vi "fit_SOS.vi"(8 "error":errorcluster, 11 "frf_data":T1) -> (0 "error out":errorcluster, 1 "return type":i32, 2 "results":dbl[](array[numeric]), 3 "theta":dbl[](array[numeric]))   [LabVIEW 2017]
uses:
  controls/SOS_frf_data.ctl
  c-src/libfit_zpk32.dll
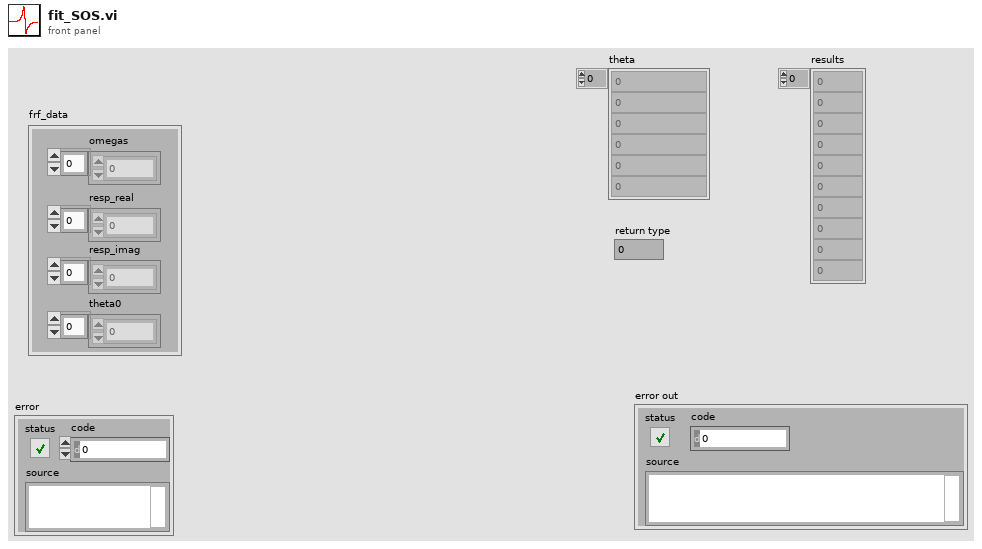
[diagram p1: front panel]
types:
  T1 = typedef "SOS_frf_data.ctl" = cluster{"omegas":dbl[], "resp_real":dbl[], "resp_imag":dbl[], "theta0":dbl[]}
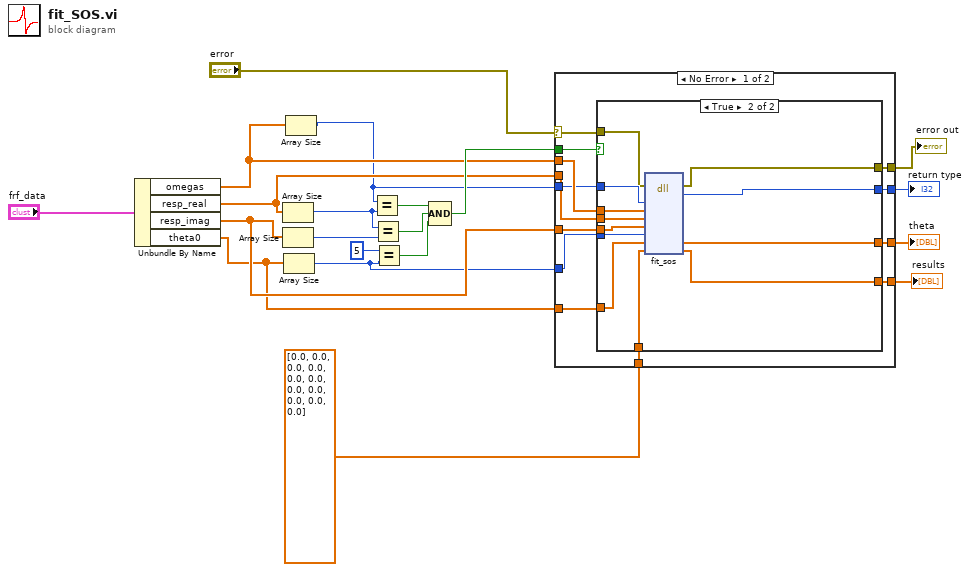
[diagram p0: block diagram]
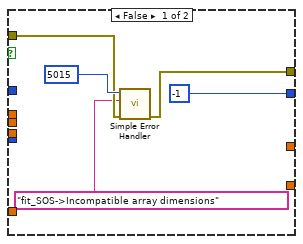
[diagram p2: hidden frame]
diagram:
  n1 = Unbundle By Name("frf_data") -> ("omegas"=w17:dbl[], "resp_real"=w16:dbl[], "resp_imag"=w15:dbl[], "theta0"=w13:dbl[])
  n2 = Array Size(array=w16) -> (size(s)=w4:i32)
  n3 = Array Size(array=w15) -> (size(s)=w5:i32)
  n4 = Array Size(array=w13) -> (size(s)=w2:i32)
  n5 = Array Size(array=w17) -> (size(s)=w6:i32)
  n6 = Equal?(x=w6, y=w4) -> (x = y?=w20:bool)
  n7 = Equal?(x=w4, y=w5) -> (x = y?=w19:bool)
  n8 = Equal?(x=5, y=w2) -> (x = y?=w1:bool)
  n9 = Compound Arithmetic op=AND(w20, w19, w1) -> (w18:bool)
  n10 = case shown="No Error" "error" {
    selector: "error" -> [w21 w51]
    tunnel: w2 -> [w33 _]
    tunnel: w18 -> [w32 _]
    tunnel: w17 -> [w31 _]
    tunnel: w16 -> [w30 _]
    tunnel: w15 -> [w29 _]
    tunnel: dbl[] [0.0, 0.0, 0.0, 0.0, 0.0, 0.0, 0.0, 0.0, 0.0, 0.0, 0.0] -> [w28 _]
    tunnel: w13 -> [w27 _]
    tunnel: [w26 _] -> w12
    tunnel: [w25 _] -> w10
    tunnel: [w24 _] -> w9
    tunnel: [w23 w51] -> w8
    tunnel: w6 -> [w22 _]
    frame No Error {
      n11 = case shown="True" w32 {
        tunnel: w27 -> [_ w50]
        tunnel: w22 -> [_ w49]
        tunnel: w33 -> [_ w48]
        tunnel: w31 -> [_ w47]
        tunnel: w30 -> [_ w46]
        tunnel: w29 -> [_ w45]
        tunnel: w28 -> [_ w44]
        tunnel: [_ w43] -> w26
        tunnel: w21 -> [w35 w42]
        tunnel: [-1 ("return type") w41] -> w25
        tunnel: [_ w40] -> w24
        tunnel: [w36 w39] -> w23
        frame False {
          n12 = call <vilib>:"Simple Error Handler.vi"("error code (no error:0)"=5015, "error source (\" \")"="fit_SOS->Incompatible array dimensions", "error in (no error)"=w35) -> ("error out"=w36:errorcluster)  [unwired: 2 in, 4 out]
        }
        frame True {
          n13 = dll-call lib="C:/Users/arnold/Documents/afm-cs/c-src/libfit_zpk32.dll" fn="fit_sos"(error in=w42, "Len_omegas"=w49, "omegas"=w47, "resp_real"=w46, "resp_imag"=w45, "len_theta"=w48, "theta"=w50, "results"=w44) -> (error out=w39:errorcluster, "return type"=w41:i32, "theta"=w43:dbl[], "results"=w40:dbl[])  [unwired: 7 in, 1 out]
        }
      }
    }
    frame Error {
    }
  }
  "theta" <- w12
  "return type" <- w10
  "results" <- w9
  "error out" <- w8
